vi "Instructor.vi"() -> ()   [LabVIEW 2017]
uses:
  <vilib>/Analysis/baseanly.llb/Mean (DBL).vi
  <vilib>/Utility/file.llb/Read Delimited Spreadsheet (DBL).vi
  <vilib>/Analysis/NI_AALBase.lvlib
panel:
  in  "TCHXActive":bool
  in  "PowerActive":bool
  in  "CTAHActive":bool
  in  "PumpActive":bool
  in  "ACTIVATE - TCHX_S":bool
  in  "ACTIVATE - PUMP_S":bool
  in  "ACTIVATE - CTAH_S":bool
  in  "Power Output On_S":bool
  in  "TCHXFreq_S":sgl format="%#.1f"
  in  "TCHXFreq":bool
  in  "Power_S":sgl format="%#.1f"
  in  "Power":bool
  in  "CTAHFreq_S":sgl format="%#.1f"
  in  "CTAHFreq":bool
  in  "PumpFreq_S":sgl format="%#.1f"
  in  "PumpFreq":bool
  out "W":sgl format="%.1f"
  out "S":sgl format="%.1f"
  out "E":sgl format="%.1f"
  out "N":sgl format="%.1f"
  out "SW":sgl format="%.1f"
  out "SE":sgl format="%.1f"
  out "N":sgl format="%.1f"
  out "Server Connection":bool
  out "Numeric":i32
  in  "B66":bool
  in  "W67":bool
  in  "B60":bool
  in  "W61":bool
  in  "B65":bool
  in  "W64":bool
  in  "B21":bool
  in  "W20":bool
  in  "B23":bool
  in  "W22":bool
  in  "B63":bool
  in  "W62":bool
  in  "A01":bool
  in  "A02":bool
  in  "W24":bool
  in  "B25":bool
  in  "W26":bool
  in  "B27":bool
  in  "B12":bool
  in  "W13":bool
  in  "C11":bool
  in  "C10":bool
  in  "S13":bool
  in  "S11":bool
  in  "S10":bool
  in  "W35":bool
  in  "B34":bool
  in  "B43":bool
  in  "W42":bool
  in  "W40":bool
  in  "B41":bool
  in  "W33":bool
  in  "B32":bool
  in  "W31":bool
  in  "B30":bool
  in  "W10":bool
  in  "B11":bool
  in  "B29":bool
  in  "W28":bool
  in  "Spoof Enabled":bool
  in  "Stop Instructor":bool
  in  "BT-63_S":sgl format="%.1g"
  in  "WT-35_S":sgl format="%.1g"
  in  "BT-34_S":sgl format="%.1g"
  in  "ST-13_S":sgl format="%.1g"
  in  "ST-11_S":sgl format="%.1g"
  in  "ST-10_S":sgl format="%.1g"
  in  "BT-29_S":sgl format="%.1g"
  in  "BT-60_S":sgl format="%.1g"
  in  "AT-02_S":sgl format="%.1g"
  in  "AT-01_S":sgl format="%.1g"
  in  "BT-30_S":sgl format="%.1g"
  in  "BT-66_S":sgl format="%.1g"
  in  "BT-65_S":sgl format="%.1g"
  in  "BT-21_S":sgl format="%.1g"
  in  "BT-23_S":sgl format="%.1g"
  in  "BT-25_S":sgl format="%.1g"
  in  "BT-27_S":sgl format="%.1g"
  in  "BT-32_S":sgl format="%.1g"
  in  "BT-43_S":sgl format="%.1g"
  in  "BT-41_S":sgl format="%.1g"
  in  "WT-67_S":sgl format="%.1g"
  in  "WT-61_S":sgl format="%.1g"
  in  "WT-64_S":sgl format="%.1g"
  in  "WT-62_S":sgl format="%.1g"
  in  "WT-20_S":sgl format="%.1g"
  in  "WT-22_S":sgl format="%.1g"
  in  "WT-33_S":sgl format="%.1g"
  in  "WT-24_S":sgl format="%.1g"
  in  "WT-26_S":sgl format="%.1g"
  in  "WT-28_S":sgl format="%.1g"
  in  "WT-42_S":sgl format="%.1g"
  in  "WT-40_S":sgl format="%.1g"
  in  "WT-31_S":sgl format="%.1g"
  in  "BT-12_S":sgl format="%.1g"
  in  "BT-11_S":sgl format="%.1g"
  in  "WT-10_S":sgl format="%.1g"
  in  "CX-11_S":sgl format="%.1g"
  in  "CX-10_S":sgl format="%.1g"
  out "DRACS Flow\n\n\nFM-60 [kg/s]":sgl format="%.3f"
  out "Primary Flow\n\n\nFM-40 [kg/s]":sgl format="%.3f"
  out "Bypass Flow\n\n\nFM-30 [kg/s]":sgl format="%.3f"
  out "DHX Primary Flow\n\n\nFM-20 [kg/s]":sgl format="%.3f"
  in  "ACTIVATE - PUMP":bool
  in  "ACTIVATE - TCHX":bool
  in  "ACTIVATE - CTAH":bool
  in  "Shutdown":bool
  in  "Power Output On":bool
  out "AT-02":sgl format="%.1g"
  out "AT-01":sgl format="%.1g"
  out "ST-13":sgl format="%.1f"
  out "ST-11":sgl format="%.1f"
  out "ST-10":sgl format="%.1f"
  out "WT-67":sgl format="%.1f"
  out "BT-66":sgl format="%.1f"
  out "BT-65":sgl format="%.1f"
  out "WT-64":sgl format="%.1f"
  out "BT-63":sgl format="%.1f"
  out "WT-62":sgl format="%.1f"
  out "WT-61":sgl format="%.1f"
  out "BT-60":sgl format="%.1f"
  out "BT-43":sgl format="%.1g"
  out "WT-42":sgl format="%.1g"
  out "BT-41":sgl format="%.1g"
  out "WT-40":sgl format="%.1g"
  out "WT-35":sgl format="%.1g"
  out "BT-34":sgl format="%.1g"
  out "WT-33":sgl format="%.1g"
  out "BT-32":sgl format="%.1g"
  out "WT-31":sgl format="%.1g"
  out "BT-30":sgl format="%.1g"
  out "BT-29":sgl format="%.1f"
  out "WT-28":sgl format="%.1f"
  out "BT-27":sgl format="%.1f"
  out "WT-26":sgl format="%.1f"
  out "BT-25":sgl format="%.1f"
  out "WT-24":sgl format="%.1f"
  out "BT-23":sgl format="%.1f"
  out "WT-22":sgl format="%.1f"
  out "BT-21":sgl format="%.1f"
  out "WT-20":sgl format="%.1f"
  out "CX-11":sgl format="%.1g"
  out "CX-10":sgl format="%.1g"
  out "WT-13":sgl format="%.1g"
  out "BT-12":sgl format="%.1g"
  out "BT-11":sgl format="%.1g"
  out "WT-10":sgl format="%.1g"
  in  "Desired Power [W]":dbl
  out "Power [W]":sgl(slide) caption="Power Output [W]" scale=0.0..10000.0
  out "Frequency [Hz]":sgl(knob) scale=0.0..45.0
  out "Frequency [Hz] 3":sgl(slide) scale=0.0..60.0
  out "Frequency [Hz]":sgl(slide) scale=0.0..60.0
  in  "WT-13_S":sgl format="%.1g"
  out "Power Output":sgl(graph)
  in  "Flow Data?":bool=TRUE
  out "System Safe":bool
  in  "Exit Profile":bool
  in  "Select Operation Mode":T1(ring) caption="Select Operation Mode2"
  out "System Time [s]":sgl format="%#.1f"
  out "System Loop Time (ms)":u32
  in  "Load Power Profile":bool
  in  "Dyn. Power Profile File":path
  out "CTAH Temperatures":cluster{"CTAH Outlet":dbl, "CTAH Inlet":dbl}(graph)
  out "CTAH Outlet":dbl format="%0.2f"
  out "CTAH Inlet":dbl format="%0.2f"
  out "Core Temperatures":cluster{"Heater Inlet":dbl, "Heater Outlet":dbl}(graph)
  out "Heater Outlet":dbl format="%0.2f"
  out "Heater Inlet":dbl format="%0.2f"
  out "Profile Step":i32
  out "Power Input Signal [W]":dbl
  out "Output Current 2 [A]":dbl
  out "Output Voltage 2 [V]":dbl
  out "Output Current 1 [A]":dbl
  out "Output Voltage 1 [V]":dbl
  out "Loop Period [ms]":i64
  in  "Pump Operation Mode":i32(listbox)
  in  "TCHX Operation Mode":i32(listbox)
  in  "VFD Stop":bool
  in  "CTAH Operation Mode":i32(listbox)
  # "System Analytics"
  # "DRACS"
  # "PRIMARY"
  # "HOT DRACS"
  # "DHX TOP"
  # "TCHX"
  # "HOT LEG"
  # "DHX"
  # "COLD DRACS"
  # "ST-14"
  # "BYPASS"
  # "CTAH"
  # "ST-12"
  # "DHX BOTTOM"
  # "HEATER"
  # "COLD LEG"
  # "PUMP"
  # "Action Log"
  # "Action Log Box"
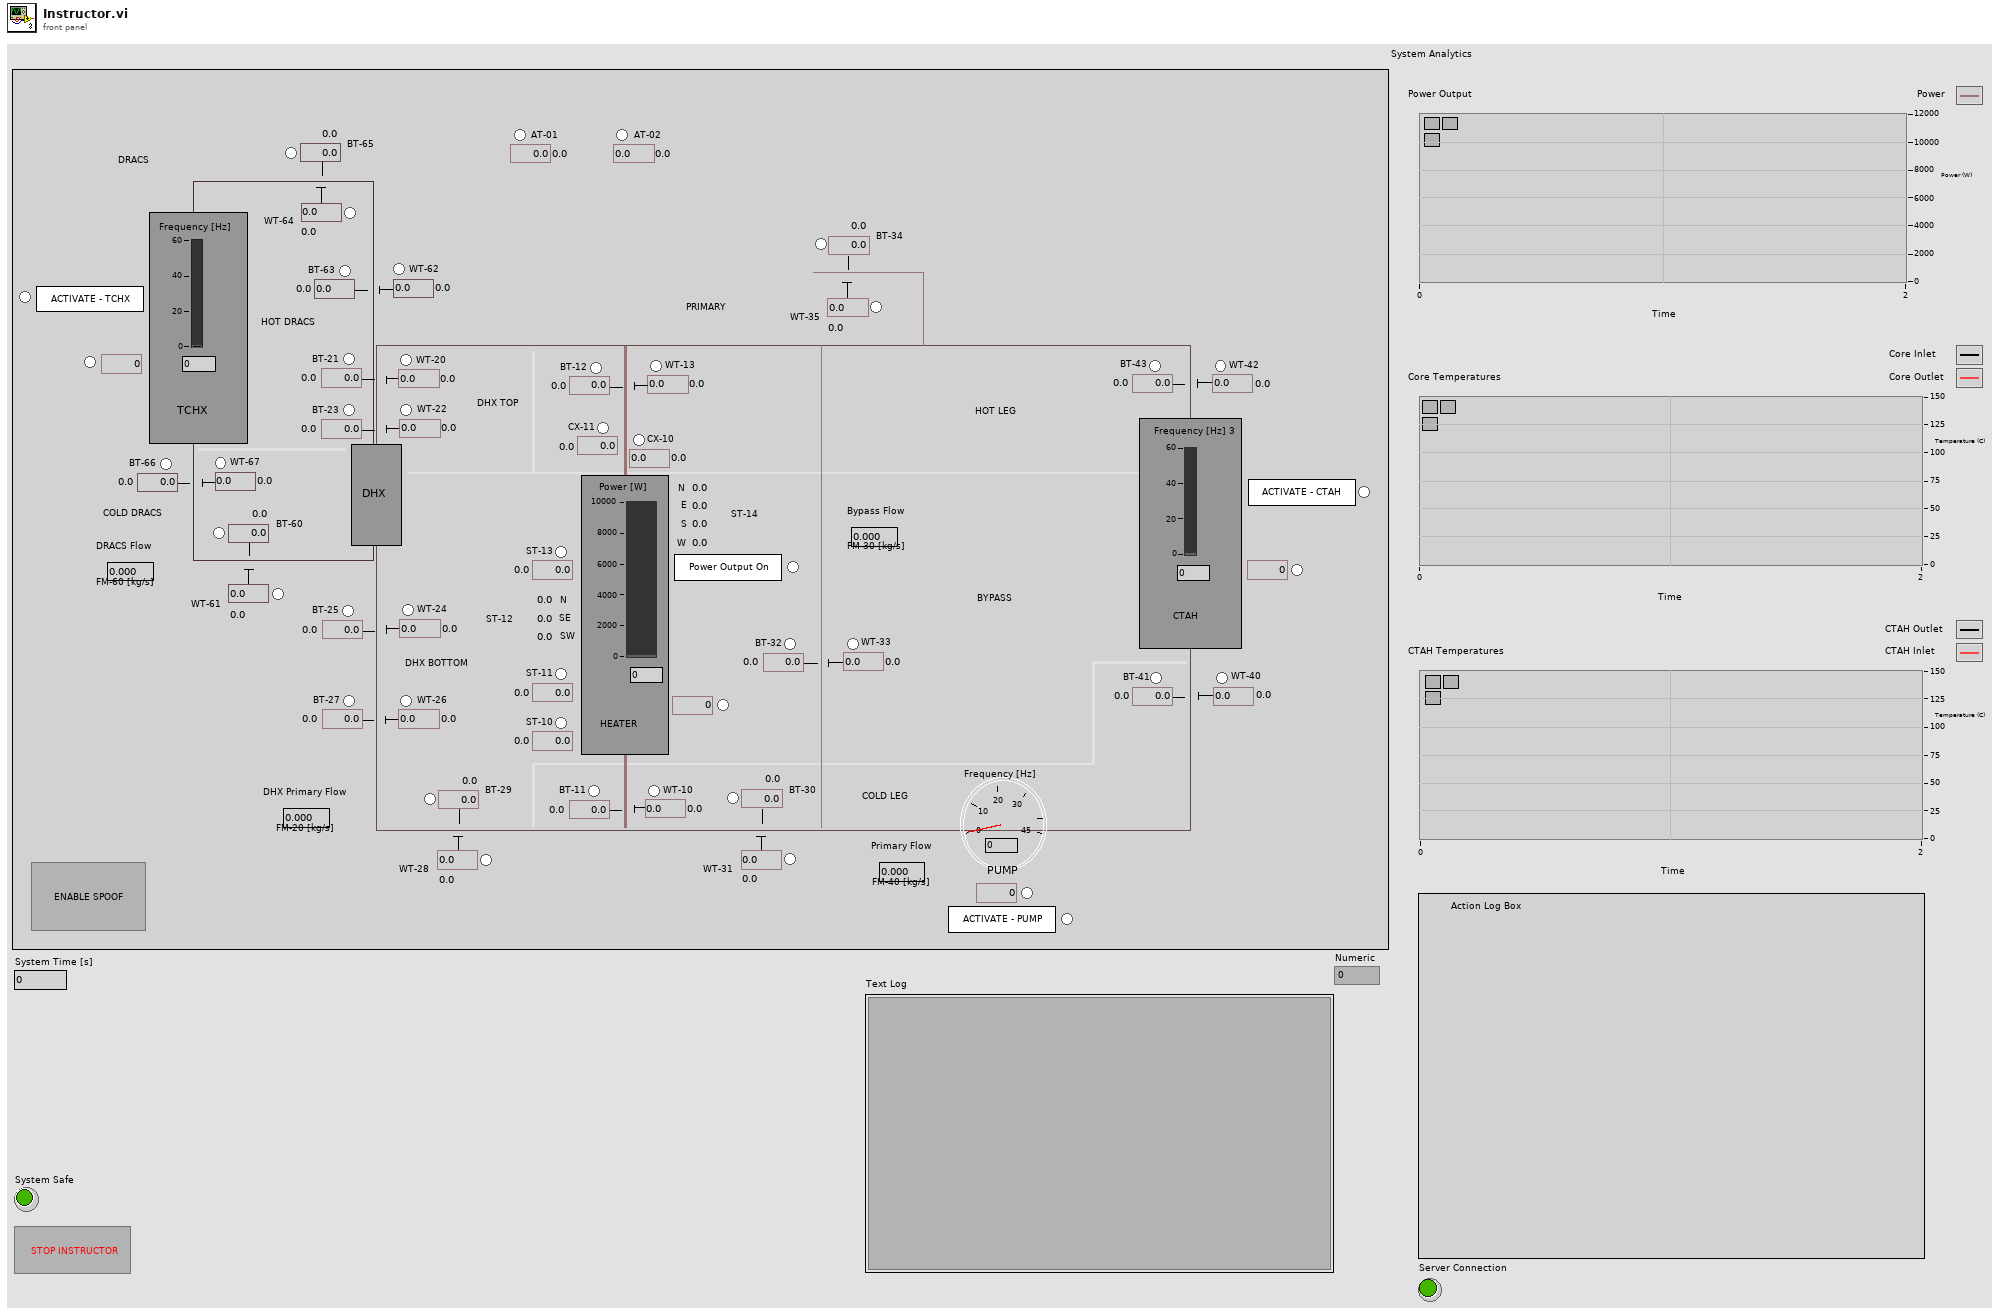
[diagram p1: front panel]
types:
  T1 = enum16{"Resistance Feedback", "Power Profile Input", "Resistance Feedback_Analog", "Power Profile Input_Analog", "Shutdown"}
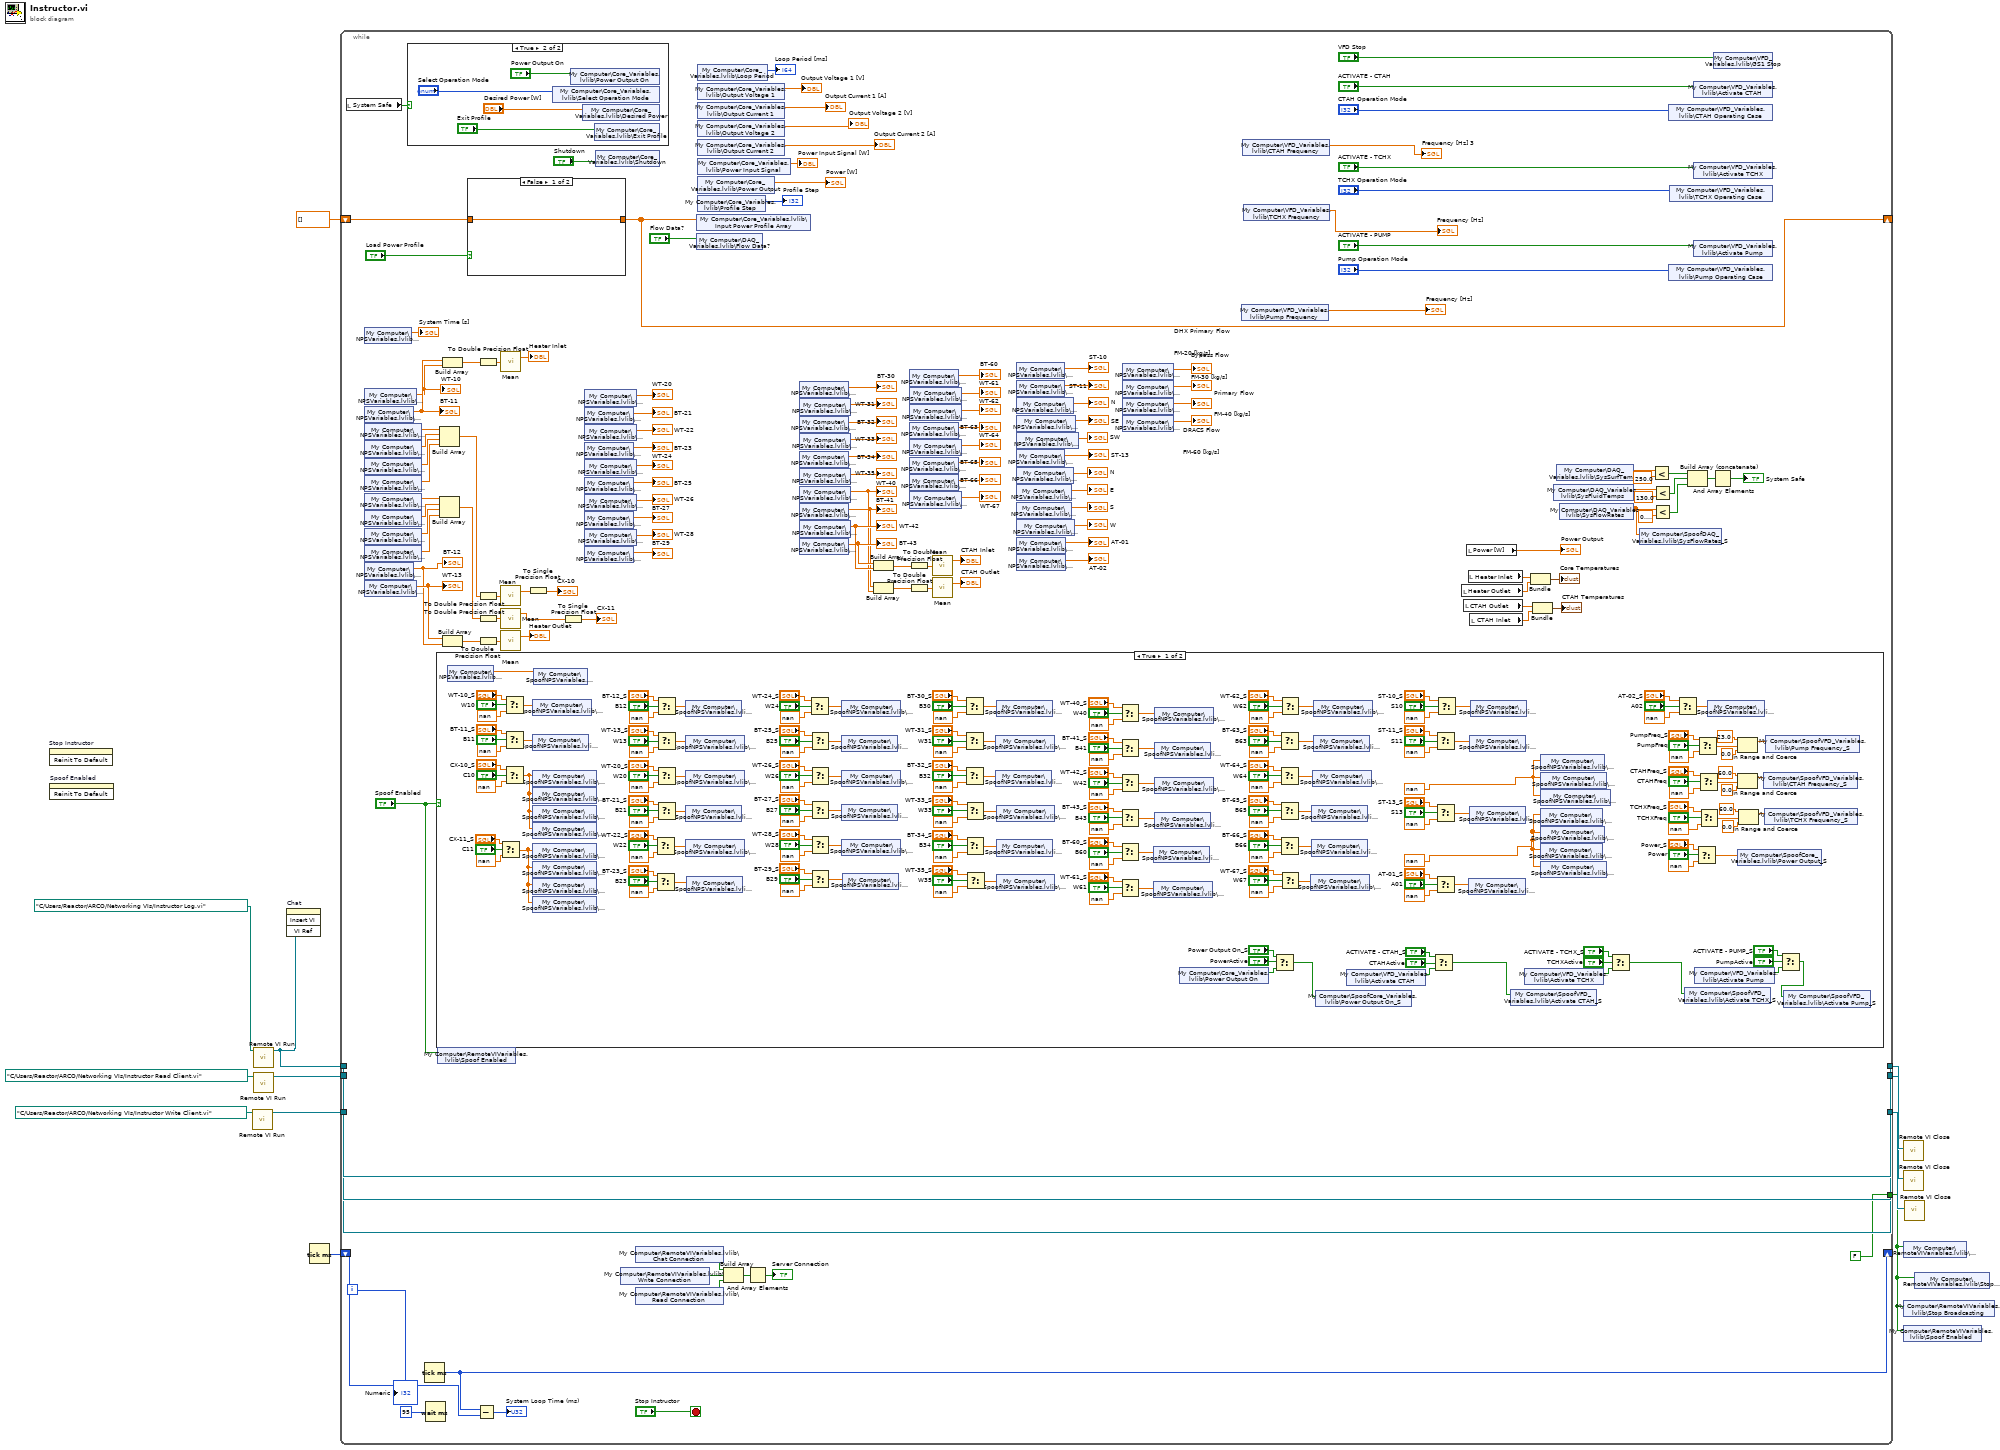
[diagram p0: block diagram]
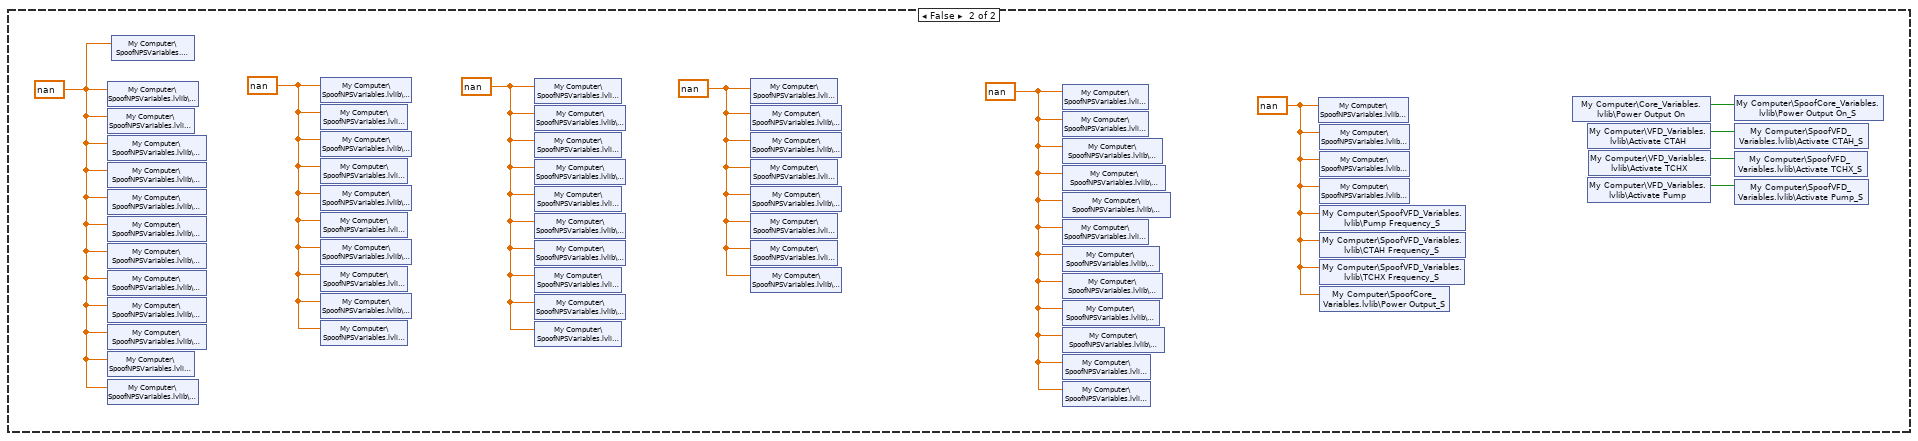
[diagram p2: hidden frame]
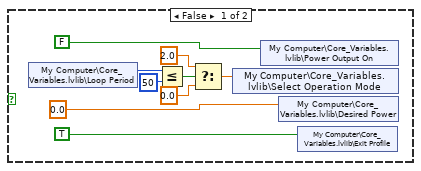
[diagram p3: hidden frame]
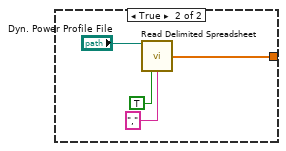
[diagram p4: hidden frame]
diagram:
  n1 = invoke on="Stop Instructor" class="Bool (strict)" method="Reinit To Default"() -> ()  [unwired: 3 in, 3 out]
  n2 = invoke on="Spoof Enabled" class="Bool (strict)" method="Reinit To Default"() -> ()  [unwired: 3 in, 3 out]
  n3 = call "Remote VI Run.vi"("VI Path"=path "C:/Users/Reactor/ARCO/Networking VIs/Instructor Write Client.vi") -> ("VI Reference"=w3:refnum<vi>)  [unwired: 10 in]
  n4 = call "Remote VI Run.vi"("VI Path"=path "C:/Users/Reactor/ARCO/Networking VIs/Instructor Log.vi" ("vi path")) -> ("VI Reference"=w9:refnum<vi>)  [unwired: 10 in]
  n5 = call "Remote VI Run.vi"("VI Path"=path "C:/Users/Reactor/ARCO/Networking VIs/Instructor Read Client.vi") -> ("VI Reference"=w7:refnum<vi>)  [unwired: 10 in]
  n6 = invoke on="Chat" class="SubPnl" method="Insert VI"("VI Ref"=w9) -> ()  [unwired: 3 in, 4 out]
  n7 = Tick Count (ms)() -> (millisecond timer value=w11:u32)
  n8 = while {
    shift-right: [w65] -> _
    shift-left: dbl[] [] ("Input Power Profile Array") -> [w66]
    shift-right: [w63] -> _
    shift-left: w11 -> [w64]
    tunnel: w9 -> [w34]
    tunnel: w7 -> [w33]
    tunnel: [w34] -> w6
    tunnel: [w33] -> w5
    tunnel: w3 -> [w32]
    tunnel: [w32] -> w2
    tunnel: [FALSE] -> w1
    i -> [w30]
    stop <- "Stop Instructor" stop-if-true
    n9 = local read "System Safe"() -> (w51:bool)
    n10 = shared-variable "My Computer\\NPSVariables.lvlib\\Time"() -> (→"System Time [s]":sgl)  [unwired: 1 in, 1 out]
    n11 = shared-variable "My Computer\\NPSVariables.lvlib\\WT-10"() -> (w41:sgl)  [unwired: 1 in, 1 out]
    "WT-10" <- w41
    n12 = shared-variable "My Computer\\NPSVariables.lvlib\\BT-11"() -> (w45:sgl)  [unwired: 1 in, 1 out]
    "BT-11" <- w45
    n13 = shared-variable "My Computer\\NPSVariables.lvlib\\CX-10-1"() -> (w131:sgl)  [unwired: 1 in, 1 out]
    n14 = shared-variable "My Computer\\NPSVariables.lvlib\\CX-10-2"() -> (w130:sgl)  [unwired: 1 in, 1 out]
    n15 = shared-variable "My Computer\\NPSVariables.lvlib\\CX-10-3"() -> (w129:sgl)  [unwired: 1 in, 1 out]
    n16 = shared-variable "My Computer\\NPSVariables.lvlib\\CX-10-4"() -> (w128:sgl)  [unwired: 1 in, 1 out]
    n17 = shared-variable "My Computer\\NPSVariables.lvlib\\CX-11-1"() -> (w124:sgl)  [unwired: 1 in, 1 out]
    n18 = shared-variable "My Computer\\NPSVariables.lvlib\\CX-11-2"() -> (w123:sgl)  [unwired: 1 in, 1 out]
    n19 = shared-variable "My Computer\\NPSVariables.lvlib\\CX-11-3"() -> (w122:sgl)  [unwired: 1 in, 1 out]
    n20 = shared-variable "My Computer\\NPSVariables.lvlib\\CX-11-4"() -> (w121:sgl)  [unwired: 1 in, 1 out]
    n21 = shared-variable "My Computer\\NPSVariables.lvlib\\BT-12"() -> (w44:sgl)  [unwired: 1 in, 1 out]
    "BT-12" <- w44
    n22 = shared-variable "My Computer\\NPSVariables.lvlib\\WT-13"() -> (w88:sgl)  [unwired: 1 in, 1 out]
    "WT-13" <- w88
    n23 = case shown="True" w51 {
      frame False {
        n24 = shared-variable "My Computer\\Core_Variables.lvlib\\Loop Period"() -> (w362:i64)  [unwired: 1 in, 1 out]
        n25 = Less Or Equal?(x=w362, y=i64 50) -> (x <= y?=w363:bool)
        n26 = Select(t=2.0, s=w363, f=0.0) -> (s? t:f=w358:dbl)
        n27 = shared-variable "My Computer\\Core_Variables.lvlib\\Select Operation Mode"(w358) -> ()  [unwired: 1 in, 1 out]
        n28 = shared-variable "My Computer\\Core_Variables.lvlib\\Power Output On"(FALSE ("Power Output On")) -> ()  [unwired: 1 in, 1 out]
        n29 = shared-variable "My Computer\\Core_Variables.lvlib\\Desired Power"(0.0 ("Desired Power")) -> ()  [unwired: 1 in, 1 out]
        n30 = shared-variable "My Computer\\Core_Variables.lvlib\\Exit Profile"(TRUE ("Exit Profile")) -> ()  [unwired: 1 in, 1 out]
      }
      frame True {
        n31 = shared-variable "My Computer\\Core_Variables.lvlib\\Select Operation Mode"("Select Operation Mode") -> ()  [unwired: 1 in, 1 out]
        n32 = shared-variable "My Computer\\Core_Variables.lvlib\\Power Output On"("Power Output On") -> ()  [unwired: 1 in, 1 out]
        n33 = shared-variable "My Computer\\Core_Variables.lvlib\\Desired Power"("Desired Power [W]") -> ()  [unwired: 1 in, 1 out]
        n34 = shared-variable "My Computer\\Core_Variables.lvlib\\Exit Profile"("Exit Profile") -> ()  [unwired: 1 in, 1 out]
      }
    }
    n35 = Tick Count (ms)() -> (millisecond timer value=w63:u32)
    n36 = Wait (ms)(milliseconds to wait=u32 95) -> ()  [unwired: 1 out]
    n37 = case shown="True" "Spoof Enabled" {
      frame True {
        w189 = sgl nan
        w190 = sgl nan
        n38 = shared-variable "My Computer\\NPSVariables.lvlib\\Time"() -> (w191:sgl)  [unwired: 1 in, 1 out]
        n39 = Select(t="CX-11_S", s="C11", f=sgl nan) -> (s? t:f=w332:sgl)
        n40 = Select(t="WT-10_S", s="W10", f=sgl nan) -> (s? t:f=w344:sgl)
        n41 = Select(t="BT-11_S", s="B11", f=sgl nan) -> (s? t:f=w340:sgl)
        n42 = Select(t="CX-10_S", s="C10", f=sgl nan) -> (s? t:f=w336:sgl)
        n43 = shared-variable "My Computer\\SpoofNPSVariables.lvlib\\WT-10_S"(w344) -> ()  [unwired: 1 in, 1 out]
        n44 = shared-variable "My Computer\\SpoofNPSVariables.lvlib\\BT-11_S"(w340) -> ()  [unwired: 1 in, 1 out]
        n45 = shared-variable "My Computer\\SpoofNPSVariables.lvlib\\CX-10-1_S"(w336) -> ()  [unwired: 1 in, 1 out]
        n46 = shared-variable "My Computer\\SpoofNPSVariables.lvlib\\CX-10-2_S"(w336) -> ()  [unwired: 1 in, 1 out]
        n47 = shared-variable "My Computer\\SpoofNPSVariables.lvlib\\CX-10-3_S"(w336) -> ()  [unwired: 1 in, 1 out]
        n48 = shared-variable "My Computer\\SpoofNPSVariables.lvlib\\CX-10-4_S"(w336) -> ()  [unwired: 1 in, 1 out]
        n49 = shared-variable "My Computer\\SpoofNPSVariables.lvlib\\CX-11-1_S"(w332) -> ()  [unwired: 1 in, 1 out]
        n50 = shared-variable "My Computer\\SpoofNPSVariables.lvlib\\CX-11-2_S"(w332) -> ()  [unwired: 1 in, 1 out]
        n51 = shared-variable "My Computer\\SpoofNPSVariables.lvlib\\CX-11-3_S"(w332) -> ()  [unwired: 1 in, 1 out]
        n52 = shared-variable "My Computer\\SpoofNPSVariables.lvlib\\CX-11-4_S"(w332) -> ()  [unwired: 1 in, 1 out]
        n53 = shared-variable "My Computer\\SpoofNPSVariables.lvlib\\Time_S"(w191) -> ()  [unwired: 1 in, 1 out]
        n54 = Select(t="WT-22_S", s="W22", f=sgl nan) -> (s? t:f=w312:sgl)
        n55 = Select(t="BT-23_S", s="B23", f=sgl nan) -> (s? t:f=w308:sgl)
        n56 = Select(t="BT-12_S", s="B12", f=sgl nan) -> (s? t:f=w328:sgl)
        n57 = Select(t="WT-13_S", s="W13", f=sgl nan) -> (s? t:f=w324:sgl)
        n58 = Select(t="WT-20_S", s="W20", f=sgl nan) -> (s? t:f=w320:sgl)
        n59 = Select(t="BT-21_S", s="B21", f=sgl nan) -> (s? t:f=w316:sgl)
        n60 = shared-variable "My Computer\\SpoofNPSVariables.lvlib\\BT-12_S"(w328) -> ()  [unwired: 1 in, 1 out]
        n61 = shared-variable "My Computer\\SpoofNPSVariables.lvlib\\WT-13_S"(w324) -> ()  [unwired: 1 in, 1 out]
        n62 = shared-variable "My Computer\\SpoofNPSVariables.lvlib\\WT-20_S"(w320) -> ()  [unwired: 1 in, 1 out]
        n63 = shared-variable "My Computer\\SpoofNPSVariables.lvlib\\BT-21_S"(w316) -> ()  [unwired: 1 in, 1 out]
        n64 = shared-variable "My Computer\\SpoofNPSVariables.lvlib\\WT-22_S"(w312) -> ()  [unwired: 1 in, 1 out]
        n65 = shared-variable "My Computer\\SpoofNPSVariables.lvlib\\BT-23_S"(w308) -> ()  [unwired: 1 in, 1 out]
        n66 = Select(t="WT-24_S", s="W24", f=sgl nan) -> (s? t:f=w304:sgl)
        n67 = Select(t="BT-25_S", s="B25", f=sgl nan) -> (s? t:f=w300:sgl)
        n68 = Select(t="WT-26_S", s="W26", f=sgl nan) -> (s? t:f=w296:sgl)
        n69 = Select(t="BT-27_S", s="B27", f=sgl nan) -> (s? t:f=w292:sgl)
        n70 = Select(t="WT-28_S", s="W28", f=sgl nan) -> (s? t:f=w288:sgl)
        n71 = Select(t="BT-29_S", s="B29", f=sgl nan) -> (s? t:f=w284:sgl)
        n72 = shared-variable "My Computer\\SpoofNPSVariables.lvlib\\WT-24_S"(w304) -> ()  [unwired: 1 in, 1 out]
        n73 = shared-variable "My Computer\\SpoofNPSVariables.lvlib\\BT-25_S"(w300) -> ()  [unwired: 1 in, 1 out]
        n74 = shared-variable "My Computer\\SpoofNPSVariables.lvlib\\WT-26_S"(w296) -> ()  [unwired: 1 in, 1 out]
        n75 = shared-variable "My Computer\\SpoofNPSVariables.lvlib\\BT-27_S"(w292) -> ()  [unwired: 1 in, 1 out]
        n76 = shared-variable "My Computer\\SpoofNPSVariables.lvlib\\WT-28_S"(w288) -> ()  [unwired: 1 in, 1 out]
        n77 = shared-variable "My Computer\\SpoofNPSVariables.lvlib\\BT-29_S"(w284) -> ()  [unwired: 1 in, 1 out]
        n78 = Select(t="BT-30_S", s="B30", f=sgl nan) -> (s? t:f=w280:sgl)
        n79 = Select(t="WT-31_S", s="W31", f=sgl nan) -> (s? t:f=w276:sgl)
        n80 = Select(t="BT-32_S", s="B32", f=sgl nan) -> (s? t:f=w272:sgl)
        n81 = Select(t="WT-33_S", s="W33", f=sgl nan) -> (s? t:f=w268:sgl)
        n82 = Select(t="BT-34_S", s="B34", f=sgl nan) -> (s? t:f=w264:sgl)
        n83 = Select(t="WT-35_S", s="W35", f=sgl nan) -> (s? t:f=w260:sgl)
        n84 = shared-variable "My Computer\\SpoofNPSVariables.lvlib\\WT-31_S"(w276) -> ()  [unwired: 1 in, 1 out]
        n85 = shared-variable "My Computer\\SpoofNPSVariables.lvlib\\BT-32_S"(w272) -> ()  [unwired: 1 in, 1 out]
        n86 = shared-variable "My Computer\\SpoofNPSVariables.lvlib\\BT-30_S"(w280) -> ()  [unwired: 1 in, 1 out]
        n87 = shared-variable "My Computer\\SpoofNPSVariables.lvlib\\WT-33_S"(w268) -> ()  [unwired: 1 in, 1 out]
        n88 = shared-variable "My Computer\\SpoofNPSVariables.lvlib\\BT-34_S"(w264) -> ()  [unwired: 1 in, 1 out]
        n89 = shared-variable "My Computer\\SpoofNPSVariables.lvlib\\WT-35_S"(w260) -> ()  [unwired: 1 in, 1 out]
        n90 = Select(t="WT-40_S", s="W40", f=sgl nan) -> (s? t:f=w256:sgl)
        n91 = Select(t="BT-41_S", s="B41", f=sgl nan) -> (s? t:f=w252:sgl)
        n92 = Select(t="WT-42_S", s="W42", f=sgl nan) -> (s? t:f=w248:sgl)
        n93 = Select(t="BT-43_S", s="B43", f=sgl nan) -> (s? t:f=w244:sgl)
        n94 = Select(t="BT-60_S", s="B60", f=sgl nan) -> (s? t:f=w240:sgl)
        n95 = Select(t="WT-61_S", s="W61", f=sgl nan) -> (s? t:f=w236:sgl)
        n96 = shared-variable "My Computer\\SpoofNPSVariables.lvlib\\BT-60_S"(w240) -> ()  [unwired: 1 in, 1 out]
        n97 = shared-variable "My Computer\\SpoofNPSVariables.lvlib\\WT-61_S"(w236) -> ()  [unwired: 1 in, 1 out]
        n98 = shared-variable "My Computer\\SpoofNPSVariables.lvlib\\BT-41_S"(w252) -> ()  [unwired: 1 in, 1 out]
        n99 = shared-variable "My Computer\\SpoofNPSVariables.lvlib\\WT-42_S"(w248) -> ()  [unwired: 1 in, 1 out]
        n100 = shared-variable "My Computer\\SpoofNPSVariables.lvlib\\BT-43_S"(w244) -> ()  [unwired: 1 in, 1 out]
        n101 = shared-variable "My Computer\\SpoofNPSVariables.lvlib\\WT-40_S"(w256) -> ()  [unwired: 1 in, 1 out]
        n102 = shared-variable "My Computer\\Core_Variables.lvlib\\Power Output On"() -> (w161:bool)  [unwired: 1 in, 1 out]
        n103 = Select(t="Power Output On_S", s="PowerActive", f=w161) -> (s? t:f=w151:bool)
        n104 = Select(t="BT-63_S", s="B63", f=sgl nan) -> (s? t:f=w228:sgl)
        n105 = Select(t="WT-64_S", s="W64", f=sgl nan) -> (s? t:f=w224:sgl)
        n106 = Select(t="BT-65_S", s="B65", f=sgl nan) -> (s? t:f=w220:sgl)
        n107 = Select(t="BT-66_S", s="B66", f=sgl nan) -> (s? t:f=w216:sgl)
        n108 = Select(t="WT-62_S", s="W62", f=sgl nan) -> (s? t:f=w232:sgl)
        n109 = Select(t="WT-67_S", s="W67", f=sgl nan) -> (s? t:f=w212:sgl)
        n110 = shared-variable "My Computer\\SpoofNPSVariables.lvlib\\WT-67_S"(w212) -> ()  [unwired: 1 in, 1 out]
        n111 = shared-variable "My Computer\\SpoofNPSVariables.lvlib\\BT-66_S"(w216) -> ()  [unwired: 1 in, 1 out]
        n112 = shared-variable "My Computer\\SpoofNPSVariables.lvlib\\BT-65_S"(w220) -> ()  [unwired: 1 in, 1 out]
        n113 = shared-variable "My Computer\\SpoofNPSVariables.lvlib\\WT-64_S"(w224) -> ()  [unwired: 1 in, 1 out]
        n114 = shared-variable "My Computer\\SpoofNPSVariables.lvlib\\BT-63_S"(w228) -> ()  [unwired: 1 in, 1 out]
        n115 = shared-variable "My Computer\\SpoofNPSVariables.lvlib\\WT-62_S"(w232) -> ()  [unwired: 1 in, 1 out]
        n116 = shared-variable "My Computer\\SpoofCore_Variables.lvlib\\Power Output On_S"(w151) -> ()  [unwired: 1 in, 1 out]
        n117 = shared-variable "My Computer\\VFD_Variables.lvlib\\Activate CTAH"() -> (w158:bool)  [unwired: 1 in, 1 out]
        n118 = Select(t="ACTIVATE - CTAH_S", s="CTAHActive", f=w158) -> (s? t:f=w150:bool)
        n119 = Select(t="ST-11_S", s="S11", f=sgl nan) -> (s? t:f=w204:sgl)
        n120 = Select(t="ST-13_S", s="S13", f=sgl nan) -> (s? t:f=w200:sgl)
        n121 = Select(t="AT-01_S", s="A01", f=sgl nan) -> (s? t:f=w196:sgl)
        n122 = Select(t="ST-10_S", s="S10", f=sgl nan) -> (s? t:f=w208:sgl)
        n123 = shared-variable "My Computer\\SpoofNPSVariables.lvlib\\AT-01_S"(w196) -> ()  [unwired: 1 in, 1 out]
        n124 = shared-variable "My Computer\\SpoofNPSVariables.lvlib\\ST-11_S"(w204) -> ()  [unwired: 1 in, 1 out]
        n125 = shared-variable "My Computer\\SpoofNPSVariables.lvlib\\ST-13_S"(w200) -> ()  [unwired: 1 in, 1 out]
        n126 = shared-variable "My Computer\\SpoofNPSVariables.lvlib\\ST-10_S"(w208) -> ()  [unwired: 1 in, 1 out]
        n127 = shared-variable "My Computer\\SpoofVFD_Variables.lvlib\\Activate CTAH_S"(w150) -> ()  [unwired: 1 in, 1 out]
        n128 = shared-variable "My Computer\\VFD_Variables.lvlib\\Activate TCHX"() -> (w155:bool)  [unwired: 1 in, 1 out]
        n129 = shared-variable "My Computer\\SpoofNPSVariables.lvlib\\ST-12-N_S"(w190) -> ()  [unwired: 1 in, 1 out]
        n130 = shared-variable "My Computer\\SpoofNPSVariables.lvlib\\ST-12-SE_S"(w190) -> ()  [unwired: 1 in, 1 out]
        n131 = shared-variable "My Computer\\SpoofNPSVariables.lvlib\\ST-12-SW_S"(w190) -> ()  [unwired: 1 in, 1 out]
        n132 = shared-variable "My Computer\\SpoofNPSVariables.lvlib\\ST-14-E_S"(w189) -> ()  [unwired: 1 in, 1 out]
        n133 = shared-variable "My Computer\\SpoofNPSVariables.lvlib\\ST-14-N_S"(w189) -> ()  [unwired: 1 in, 1 out]
        n134 = shared-variable "My Computer\\SpoofNPSVariables.lvlib\\ST-14-S_S"(w189) -> ()  [unwired: 1 in, 1 out]
        n135 = shared-variable "My Computer\\SpoofNPSVariables.lvlib\\ST-14-W_S"(w189) -> ()  [unwired: 1 in, 1 out]
        n136 = Select(t="ACTIVATE - TCHX_S", s="TCHXActive", f=w155) -> (s? t:f=w148:bool)
        n137 = Select(t="AT-02_S", s="A02", f=sgl nan) -> (s? t:f=w192:sgl)
        n138 = shared-variable "My Computer\\SpoofVFD_Variables.lvlib\\Activate TCHX_S"(w148) -> ()  [unwired: 1 in, 1 out]
        n139 = shared-variable "My Computer\\VFD_Variables.lvlib\\Activate Pump"() -> (w152:bool)  [unwired: 1 in, 1 out]
        n140 = Select(t="Power_S", s="Power", f=sgl nan) -> (s? t:f=w164:sgl)
        n141 = Select(t="PumpFreq_S", s="PumpFreq", f=sgl nan) -> (s? t:f=w183:sgl)
        n142 = Select(t="CTAHFreq_S", s="CTAHFreq", f=sgl nan) -> (s? t:f=w179:sgl)
        n143 = Select(t="TCHXFreq_S", s="TCHXFreq", f=sgl nan) -> (s? t:f=w172:sgl)
        n144 = shared-variable "My Computer\\SpoofNPSVariables.lvlib\\AT-02_S"(w192) -> ()  [unwired: 1 in, 1 out]
        n145 = In Range and Coerce(upper limit=sgl 23.0, x=w183, lower limit=sgl 0.0) -> (coerced(x)=w182:sgl)  [unwired: 1 out]
        n146 = shared-variable "My Computer\\SpoofCore_Variables.lvlib\\Power Output_S"(w164) -> ()  [unwired: 1 in, 1 out]
        n147 = In Range and Coerce(upper limit=sgl 60.0, x=w179, lower limit=sgl 0.0) -> (coerced(x)=w175:sgl)  [unwired: 1 out]
        n148 = In Range and Coerce(upper limit=sgl 60.0, x=w172, lower limit=sgl 0.0) -> (coerced(x)=w168:sgl)  [unwired: 1 out]
        n149 = shared-variable "My Computer\\SpoofVFD_Variables.lvlib\\CTAH Frequency_S"(w175) -> ()  [unwired: 1 in, 1 out]
        n150 = shared-variable "My Computer\\SpoofVFD_Variables.lvlib\\TCHX Frequency_S"(w168) -> ()  [unwired: 1 in, 1 out]
        n151 = shared-variable "My Computer\\SpoofVFD_Variables.lvlib\\Pump Frequency_S"(w182) -> ()  [unwired: 1 in, 1 out]
        n152 = Select(t="ACTIVATE - PUMP_S", s="PumpActive", f=w152) -> (s? t:f=w149:bool)
        n153 = shared-variable "My Computer\\SpoofVFD_Variables.lvlib\\Activate Pump_S"(w149) -> ()  [unwired: 1 in, 1 out]
      }
      frame False {
        w352 = sgl nan
        w354 = sgl nan
        w355 = sgl nan
        w356 = sgl nan
        w357 = sgl nan
        w353 = sgl nan
        n154 = shared-variable "My Computer\\SpoofNPSVariables.lvlib\\WT-10_S"(w353) -> ()  [unwired: 1 in, 1 out]
        n155 = shared-variable "My Computer\\SpoofNPSVariables.lvlib\\BT-11_S"(w353) -> ()  [unwired: 1 in, 1 out]
        n156 = shared-variable "My Computer\\SpoofNPSVariables.lvlib\\CX-10-1_S"(w353) -> ()  [unwired: 1 in, 1 out]
        n157 = shared-variable "My Computer\\SpoofNPSVariables.lvlib\\CX-10-2_S"(w353) -> ()  [unwired: 1 in, 1 out]
        n158 = shared-variable "My Computer\\SpoofNPSVariables.lvlib\\CX-10-3_S"(w353) -> ()  [unwired: 1 in, 1 out]
        n159 = shared-variable "My Computer\\SpoofNPSVariables.lvlib\\CX-10-4_S"(w353) -> ()  [unwired: 1 in, 1 out]
        n160 = shared-variable "My Computer\\SpoofNPSVariables.lvlib\\CX-11-1_S"(w353) -> ()  [unwired: 1 in, 1 out]
        n161 = shared-variable "My Computer\\SpoofNPSVariables.lvlib\\CX-11-2_S"(w353) -> ()  [unwired: 1 in, 1 out]
        n162 = shared-variable "My Computer\\SpoofNPSVariables.lvlib\\CX-11-3_S"(w353) -> ()  [unwired: 1 in, 1 out]
        n163 = shared-variable "My Computer\\SpoofNPSVariables.lvlib\\CX-11-4_S"(w353) -> ()  [unwired: 1 in, 1 out]
        n164 = shared-variable "My Computer\\SpoofNPSVariables.lvlib\\BT-12_S"(w353) -> ()  [unwired: 1 in, 1 out]
        n165 = shared-variable "My Computer\\SpoofNPSVariables.lvlib\\WT-13_S"(w353) -> ()  [unwired: 1 in, 1 out]
        n166 = shared-variable "My Computer\\SpoofNPSVariables.lvlib\\Time_S"(w353) -> ()  [unwired: 1 in, 1 out]
        n167 = shared-variable "My Computer\\SpoofNPSVariables.lvlib\\WT-20_S"(w357) -> ()  [unwired: 1 in, 1 out]
        n168 = shared-variable "My Computer\\SpoofNPSVariables.lvlib\\BT-21_S"(w357) -> ()  [unwired: 1 in, 1 out]
        n169 = shared-variable "My Computer\\SpoofNPSVariables.lvlib\\WT-22_S"(w357) -> ()  [unwired: 1 in, 1 out]
        n170 = shared-variable "My Computer\\SpoofNPSVariables.lvlib\\BT-23_S"(w357) -> ()  [unwired: 1 in, 1 out]
        n171 = shared-variable "My Computer\\SpoofNPSVariables.lvlib\\WT-24_S"(w357) -> ()  [unwired: 1 in, 1 out]
        n172 = shared-variable "My Computer\\SpoofNPSVariables.lvlib\\BT-25_S"(w357) -> ()  [unwired: 1 in, 1 out]
        n173 = shared-variable "My Computer\\SpoofNPSVariables.lvlib\\WT-26_S"(w357) -> ()  [unwired: 1 in, 1 out]
        n174 = shared-variable "My Computer\\SpoofNPSVariables.lvlib\\BT-27_S"(w357) -> ()  [unwired: 1 in, 1 out]
        n175 = shared-variable "My Computer\\SpoofNPSVariables.lvlib\\WT-28_S"(w357) -> ()  [unwired: 1 in, 1 out]
        n176 = shared-variable "My Computer\\SpoofNPSVariables.lvlib\\BT-29_S"(w357) -> ()  [unwired: 1 in, 1 out]
        n177 = shared-variable "My Computer\\SpoofNPSVariables.lvlib\\BT-30_S"(w356) -> ()  [unwired: 1 in, 1 out]
        n178 = shared-variable "My Computer\\SpoofNPSVariables.lvlib\\WT-31_S"(w356) -> ()  [unwired: 1 in, 1 out]
        n179 = shared-variable "My Computer\\SpoofNPSVariables.lvlib\\BT-32_S"(w356) -> ()  [unwired: 1 in, 1 out]
        n180 = shared-variable "My Computer\\SpoofNPSVariables.lvlib\\WT-33_S"(w356) -> ()  [unwired: 1 in, 1 out]
        n181 = shared-variable "My Computer\\SpoofNPSVariables.lvlib\\BT-34_S"(w356) -> ()  [unwired: 1 in, 1 out]
        n182 = shared-variable "My Computer\\SpoofNPSVariables.lvlib\\WT-35_S"(w356) -> ()  [unwired: 1 in, 1 out]
        n183 = shared-variable "My Computer\\SpoofNPSVariables.lvlib\\WT-40_S"(w356) -> ()  [unwired: 1 in, 1 out]
        n184 = shared-variable "My Computer\\SpoofNPSVariables.lvlib\\BT-41_S"(w356) -> ()  [unwired: 1 in, 1 out]
        n185 = shared-variable "My Computer\\SpoofNPSVariables.lvlib\\WT-42_S"(w356) -> ()  [unwired: 1 in, 1 out]
        n186 = shared-variable "My Computer\\SpoofNPSVariables.lvlib\\BT-43_S"(w356) -> ()  [unwired: 1 in, 1 out]
        n187 = shared-variable "My Computer\\SpoofNPSVariables.lvlib\\BT-60_S"(w355) -> ()  [unwired: 1 in, 1 out]
        n188 = shared-variable "My Computer\\SpoofNPSVariables.lvlib\\WT-61_S"(w355) -> ()  [unwired: 1 in, 1 out]
        n189 = shared-variable "My Computer\\SpoofNPSVariables.lvlib\\WT-62_S"(w355) -> ()  [unwired: 1 in, 1 out]
        n190 = shared-variable "My Computer\\SpoofNPSVariables.lvlib\\BT-63_S"(w355) -> ()  [unwired: 1 in, 1 out]
        n191 = shared-variable "My Computer\\SpoofNPSVariables.lvlib\\WT-64_S"(w355) -> ()  [unwired: 1 in, 1 out]
        n192 = shared-variable "My Computer\\SpoofNPSVariables.lvlib\\BT-65_S"(w355) -> ()  [unwired: 1 in, 1 out]
        n193 = shared-variable "My Computer\\SpoofNPSVariables.lvlib\\BT-66_S"(w355) -> ()  [unwired: 1 in, 1 out]
        n194 = shared-variable "My Computer\\SpoofNPSVariables.lvlib\\WT-67_S"(w355) -> ()  [unwired: 1 in, 1 out]
        n195 = shared-variable "My Computer\\SpoofNPSVariables.lvlib\\ST-10_S"(w354) -> ()  [unwired: 1 in, 1 out]
        n196 = shared-variable "My Computer\\SpoofNPSVariables.lvlib\\ST-11_S"(w354) -> ()  [unwired: 1 in, 1 out]
        n197 = shared-variable "My Computer\\SpoofNPSVariables.lvlib\\ST-12-N_S"(w354) -> ()  [unwired: 1 in, 1 out]
        n198 = shared-variable "My Computer\\SpoofNPSVariables.lvlib\\ST-12-SE_S"(w354) -> ()  [unwired: 1 in, 1 out]
        n199 = shared-variable "My Computer\\SpoofNPSVariables.lvlib\\ST-12-SW_S"(w354) -> ()  [unwired: 1 in, 1 out]
        n200 = shared-variable "My Computer\\SpoofNPSVariables.lvlib\\ST-13_S"(w354) -> ()  [unwired: 1 in, 1 out]
        n201 = shared-variable "My Computer\\SpoofNPSVariables.lvlib\\ST-14-E_S"(w354) -> ()  [unwired: 1 in, 1 out]
        n202 = shared-variable "My Computer\\SpoofNPSVariables.lvlib\\ST-14-N_S"(w354) -> ()  [unwired: 1 in, 1 out]
        n203 = shared-variable "My Computer\\SpoofNPSVariables.lvlib\\ST-14-S_S"(w354) -> ()  [unwired: 1 in, 1 out]
        n204 = shared-variable "My Computer\\SpoofNPSVariables.lvlib\\ST-14-W_S"(w354) -> ()  [unwired: 1 in, 1 out]
        n205 = shared-variable "My Computer\\SpoofNPSVariables.lvlib\\AT-01_S"(w354) -> ()  [unwired: 1 in, 1 out]
        n206 = shared-variable "My Computer\\SpoofNPSVariables.lvlib\\AT-02_S"(w354) -> ()  [unwired: 1 in, 1 out]
        n207 = shared-variable "My Computer\\SpoofNPSVariables.lvlib\\FM-20_S"(w352) -> ()  [unwired: 1 in, 1 out]
        n208 = shared-variable "My Computer\\SpoofNPSVariables.lvlib\\FM-30_S"(w352) -> ()  [unwired: 1 in, 1 out]
        n209 = shared-variable "My Computer\\SpoofNPSVariables.lvlib\\FM-40_S"(w352) -> ()  [unwired: 1 in, 1 out]
        n210 = shared-variable "My Computer\\SpoofNPSVariables.lvlib\\FM-60_S"(w352) -> ()  [unwired: 1 in, 1 out]
        n211 = shared-variable "My Computer\\SpoofVFD_Variables.lvlib\\Pump Frequency_S"(w352) -> ()  [unwired: 1 in, 1 out]
        n212 = shared-variable "My Computer\\SpoofVFD_Variables.lvlib\\CTAH Frequency_S"(w352) -> ()  [unwired: 1 in, 1 out]
        n213 = shared-variable "My Computer\\SpoofVFD_Variables.lvlib\\TCHX Frequency_S"(w352) -> ()  [unwired: 1 in, 1 out]
        n214 = shared-variable "My Computer\\SpoofCore_Variables.lvlib\\Power Output_S"(w352) -> ()  [unwired: 1 in, 1 out]
        n215 = shared-variable "My Computer\\Core_Variables.lvlib\\Power Output On"() -> (w351:bool)  [unwired: 1 in, 1 out]
        n216 = shared-variable "My Computer\\VFD_Variables.lvlib\\Activate CTAH"() -> (w350:bool)  [unwired: 1 in, 1 out]
        n217 = shared-variable "My Computer\\VFD_Variables.lvlib\\Activate Pump"() -> (w348:bool)  [unwired: 1 in, 1 out]
        n218 = shared-variable "My Computer\\VFD_Variables.lvlib\\Activate TCHX"() -> (w349:bool)  [unwired: 1 in, 1 out]
        n219 = shared-variable "My Computer\\SpoofCore_Variables.lvlib\\Power Output On_S"(w351) -> ()  [unwired: 1 in, 1 out]
        n220 = shared-variable "My Computer\\SpoofVFD_Variables.lvlib\\Activate CTAH_S"(w350) -> ()  [unwired: 1 in, 1 out]
        n221 = shared-variable "My Computer\\SpoofVFD_Variables.lvlib\\Activate TCHX_S"(w349) -> ()  [unwired: 1 in, 1 out]
        n222 = shared-variable "My Computer\\SpoofVFD_Variables.lvlib\\Activate Pump_S"(w348) -> ()  [unwired: 1 in, 1 out]
      }
    }
    n223 = shared-variable "My Computer\\RemoteVIVariables.lvlib\\Spoof Enabled"("Spoof Enabled") -> ()  [unwired: 1 in, 1 out]
    n224 = Build Array(w131, w130, w129, w128) -> (w127:sgl[])
    n225 = Build Array(w124, w123, w122, w121) -> (w120:sgl[])
    n226 = Build Array(w45, w41) -> (w86:sgl[])
    n227 = Build Array(w88, w44) -> (w89:sgl[])
    n228 = case shown="False" "Load Power Profile" {
      tunnel: [w371 w372] -> w65
      tunnel: w66 -> [w371 _]
      frame False {
      }
      frame True {
        n229 = call-poly <vilib>:"Read Delimited Spreadsheet.vi"("file path (dialog if empty)"="Dyn. Power Profile File", "transpose? (F)"=TRUE, "delimiter (\\t)"="," ("delimiter (\\t)")) -> ("first row"=w372:dbl[])  [unwired: 7 in, 5 out]
      }
    }
    n230 = Subtract(x=w63, y=w64) -> (x-y=→"System Loop Time (ms)":u32)
    n231 = To Double Precision Float(number=w86) -> (double precision float=w87:dbl[])
    n232 = To Double Precision Float(number=w127) -> (double precision float=w126:dbl[])
    n233 = To Double Precision Float(number=w120) -> (double precision float=w125:dbl[])
    n234 = To Double Precision Float(number=w89) -> (double precision float=w90:dbl[])
    n235 = call-poly <vilib>:"Mean.vi"("X"=w87) -> ("mean"=→"Heater Inlet":dbl)  [unwired: 1 out]
    n236 = call-poly <vilib>:"Mean.vi"("X"=w126) -> ("mean"=w47:dbl)  [unwired: 1 out]
    n237 = call-poly <vilib>:"Mean.vi"("X"=w125) -> ("mean"=w46:dbl)  [unwired: 1 out]
    n238 = call-poly <vilib>:"Mean.vi"("X"=w90) -> ("mean"=→"Heater Outlet":dbl)  [unwired: 1 out]
    n239 = To Single Precision Float(number=w47) -> (single precision float=→"CX-10":sgl)
    n240 = To Single Precision Float(number=w46) -> (single precision float=→"CX-11":sgl)
    n241 = shared-variable "My Computer\\NPSVariables.lvlib\\WT-20"() -> (→"WT-20":sgl)  [unwired: 1 in, 1 out]
    n242 = shared-variable "My Computer\\NPSVariables.lvlib\\BT-21"() -> (→"BT-21":sgl)  [unwired: 1 in, 1 out]
    n243 = shared-variable "My Computer\\NPSVariables.lvlib\\WT-22"() -> (→"WT-22":sgl)  [unwired: 1 in, 1 out]
    n244 = shared-variable "My Computer\\NPSVariables.lvlib\\BT-23"() -> (→"BT-23":sgl)  [unwired: 1 in, 1 out]
    n245 = shared-variable "My Computer\\NPSVariables.lvlib\\WT-24"() -> (→"WT-24":sgl)  [unwired: 1 in, 1 out]
    n246 = shared-variable "My Computer\\NPSVariables.lvlib\\BT-25"() -> (→"BT-25":sgl)  [unwired: 1 in, 1 out]
    n247 = shared-variable "My Computer\\NPSVariables.lvlib\\WT-26"() -> (→"WT-26":sgl)  [unwired: 1 in, 1 out]
    n248 = shared-variable "My Computer\\NPSVariables.lvlib\\BT-27"() -> (→"BT-27":sgl)  [unwired: 1 in, 1 out]
    n249 = shared-variable "My Computer\\NPSVariables.lvlib\\WT-28"() -> (→"WT-28":sgl)  [unwired: 1 in, 1 out]
    n250 = shared-variable "My Computer\\NPSVariables.lvlib\\BT-29"() -> (→"BT-29":sgl)  [unwired: 1 in, 1 out]
    n251 = shared-variable "My Computer\\Core_Variables.lvlib\\Shutdown"("Shutdown") -> ()  [unwired: 1 in, 1 out]
    n252 = shared-variable "My Computer\\RemoteVIVariables.lvlib\\Write Connection"() -> (w28:bool)  [unwired: 1 in, 1 out]
    n253 = shared-variable "My Computer\\RemoteVIVariables.lvlib\\Read Connection"() -> (w27:bool)  [unwired: 1 in, 1 out]
    n254 = shared-variable "My Computer\\RemoteVIVariables.lvlib\\Chat Connection"() -> (w29:bool)  [unwired: 1 in, 1 out]
    n255 = shared-variable "My Computer\\Core_Variables.lvlib\\Input Power Profile Array"(w65) -> ()  [unwired: 1 in, 1 out]
    n256 = shared-variable "My Computer\\DAQ_Variables.lvlib\\Flow Data?"("Flow Data?") -> ()  [unwired: 1 in, 1 out]
    n257 = shared-variable "My Computer\\Core_Variables.lvlib\\Loop Period"() -> (→"Loop Period [ms]":i64)  [unwired: 1 in, 1 out]
    n258 = shared-variable "My Computer\\Core_Variables.lvlib\\Output Voltage 1"() -> (→"Output Voltage 1 [V]":dbl)  [unwired: 1 in, 1 out]
    n259 = shared-variable "My Computer\\Core_Variables.lvlib\\Output Current 1"() -> (→"Output Current 1 [A]":dbl)  [unwired: 1 in, 1 out]
    n260 = shared-variable "My Computer\\Core_Variables.lvlib\\Output Voltage 2"() -> (→"Output Voltage 2 [V]":dbl)  [unwired: 1 in, 1 out]
    n261 = shared-variable "My Computer\\Core_Variables.lvlib\\Output Current 2"() -> (→"Output Current 2 [A]":dbl)  [unwired: 1 in, 1 out]
    n262 = shared-variable "My Computer\\Core_Variables.lvlib\\Power Input Signal"() -> (→"Power Input Signal [W]":sgl)  [unwired: 1 in, 1 out]
    n263 = shared-variable "My Computer\\Core_Variables.lvlib\\Power Output"() -> (→"Power [W]":sgl)  [unwired: 1 in, 1 out]
    n264 = shared-variable "My Computer\\Core_Variables.lvlib\\Profile Step"() -> (→"Profile Step":i32)  [unwired: 1 in, 1 out]
    n265 = Build Array(w29, w28, w27) -> (w26:bool[])
    n266 = And Array Elements(Boolean array=w26) -> (logical AND=→"Server Connection":bool)
    n267 = shared-variable "My Computer\\NPSVariables.lvlib\\BT-30"() -> (→"BT-30":sgl)  [unwired: 1 in, 1 out]
    n268 = shared-variable "My Computer\\NPSVariables.lvlib\\WT-31"() -> (→"WT-31":sgl)  [unwired: 1 in, 1 out]
    n269 = shared-variable "My Computer\\NPSVariables.lvlib\\BT-32"() -> (→"BT-32":sgl)  [unwired: 1 in, 1 out]
    n270 = shared-variable "My Computer\\NPSVariables.lvlib\\WT-33"() -> (→"WT-33":sgl)  [unwired: 1 in, 1 out]
    n271 = shared-variable "My Computer\\NPSVariables.lvlib\\BT-34"() -> (→"BT-34":sgl)  [unwired: 1 in, 1 out]
    n272 = shared-variable "My Computer\\NPSVariables.lvlib\\WT-35"() -> (→"WT-35":sgl)  [unwired: 1 in, 1 out]
    n273 = shared-variable "My Computer\\NPSVariables.lvlib\\WT-40"() -> (w72:sgl)  [unwired: 1 in, 1 out]
    "WT-40" <- w72
    n274 = shared-variable "My Computer\\NPSVariables.lvlib\\BT-41"() -> (w71:sgl)  [unwired: 1 in, 1 out]
    "BT-41" <- w71
    n275 = shared-variable "My Computer\\NPSVariables.lvlib\\WT-42"() -> (w74:sgl)  [unwired: 1 in, 1 out]
    "WT-42" <- w74
    n276 = shared-variable "My Computer\\NPSVariables.lvlib\\BT-43"() -> (w73:sgl)  [unwired: 1 in, 1 out]
    "BT-43" <- w73
    n277 = Build Array(w73, w74) -> (w79:sgl[])
    n278 = Build Array(w71, w72) -> (w76:sgl[])
    n279 = shared-variable "My Computer\\NPSVariables.lvlib\\BT-60"() -> (→"BT-60":sgl)  [unwired: 1 in, 1 out]
    n280 = shared-variable "My Computer\\NPSVariables.lvlib\\WT-61"() -> (→"WT-61":sgl)  [unwired: 1 in, 1 out]
    n281 = shared-variable "My Computer\\NPSVariables.lvlib\\WT-62"() -> (→"WT-62":sgl)  [unwired: 1 in, 1 out]
    n282 = shared-variable "My Computer\\NPSVariables.lvlib\\BT-63"() -> (→"BT-63":sgl)  [unwired: 1 in, 1 out]
    n283 = shared-variable "My Computer\\NPSVariables.lvlib\\WT-64"() -> (→"WT-64":sgl)  [unwired: 1 in, 1 out]
    n284 = shared-variable "My Computer\\NPSVariables.lvlib\\BT-65"() -> (→"BT-65":sgl)  [unwired: 1 in, 1 out]
    n285 = shared-variable "My Computer\\NPSVariables.lvlib\\BT-66"() -> (→"BT-66":sgl)  [unwired: 1 in, 1 out]
    n286 = shared-variable "My Computer\\NPSVariables.lvlib\\WT-67"() -> (→"WT-67":sgl)  [unwired: 1 in, 1 out]
    n287 = To Double Precision Float(number=w79) -> (double precision float=w80:dbl[])
    n288 = To Double Precision Float(number=w76) -> (double precision float=w77:dbl[])
    n289 = call-poly <vilib>:"Mean.vi"("X"=w80) -> ("mean"=→"CTAH Inlet":dbl)  [unwired: 1 out]
    n290 = call-poly <vilib>:"Mean.vi"("X"=w77) -> ("mean"=→"CTAH Outlet":dbl)  [unwired: 1 out]
    n291 = shared-variable "My Computer\\NPSVariables.lvlib\\ST-10"() -> (→"ST-10":sgl)  [unwired: 1 in, 1 out]
    n292 = shared-variable "My Computer\\NPSVariables.lvlib\\ST-11"() -> (→"ST-11":sgl)  [unwired: 1 in, 1 out]
    n293 = shared-variable "My Computer\\NPSVariables.lvlib\\ST-12-N"() -> (→"N":sgl)  [unwired: 1 in, 1 out]
    n294 = shared-variable "My Computer\\NPSVariables.lvlib\\ST-12-SE"() -> (→"SE":sgl)  [unwired: 1 in, 1 out]
    n295 = shared-variable "My Computer\\NPSVariables.lvlib\\ST-12-SW"() -> (→"SW":sgl)  [unwired: 1 in, 1 out]
    n296 = shared-variable "My Computer\\NPSVariables.lvlib\\ST-13"() -> (→"ST-13":sgl)  [unwired: 1 in, 1 out]
    n297 = shared-variable "My Computer\\NPSVariables.lvlib\\ST-14-N"() -> (→"N":sgl)  [unwired: 1 in, 1 out]
    n298 = shared-variable "My Computer\\NPSVariables.lvlib\\ST-14-E"() -> (→"E":sgl)  [unwired: 1 in, 1 out]
    n299 = shared-variable "My Computer\\NPSVariables.lvlib\\ST-14-S"() -> (→"S":sgl)  [unwired: 1 in, 1 out]
    n300 = shared-variable "My Computer\\NPSVariables.lvlib\\ST-14-W"() -> (→"W":sgl)  [unwired: 1 in, 1 out]
    n301 = shared-variable "My Computer\\NPSVariables.lvlib\\AT-01"() -> (→"AT-01":sgl)  [unwired: 1 in, 1 out]
    n302 = shared-variable "My Computer\\NPSVariables.lvlib\\AT-02"() -> (→"AT-02":sgl)  [unwired: 1 in, 1 out]
    n303 = shared-variable "My Computer\\NPSVariables.lvlib\\FM-20"() -> (→"DHX Primary Flow\n\n\nFM-20 [kg/s]":sgl)  [unwired: 1 in, 1 out]
    n304 = shared-variable "My Computer\\NPSVariables.lvlib\\FM-30"() -> (→"Bypass Flow\n\n\nFM-30 [kg/s]":sgl)  [unwired: 1 in, 1 out]
    n305 = shared-variable "My Computer\\NPSVariables.lvlib\\FM-40"() -> (→"Primary Flow\n\n\nFM-40 [kg/s]":sgl)  [unwired: 1 in, 1 out]
    n306 = shared-variable "My Computer\\NPSVariables.lvlib\\FM-60"() -> (→"DRACS Flow\n\n\nFM-60 [kg/s]":sgl)  [unwired: 1 in, 1 out]
    n307 = shared-variable "My Computer\\VFD_Variables.lvlib\\Pump Frequency"() -> (→"Frequency [Hz]":sgl)  [unwired: 1 in, 1 out]
    n308 = shared-variable "My Computer\\VFD_Variables.lvlib\\CTAH Frequency"() -> (→"Frequency [Hz] 3":sgl)  [unwired: 1 in, 1 out]
    n309 = shared-variable "My Computer\\VFD_Variables.lvlib\\TCHX Frequency"() -> (→"Frequency [Hz]":sgl)  [unwired: 1 in, 1 out]
    n310 = local read "Heater Outlet"() -> (w81:dbl)
    n311 = local read "CTAH Outlet"() -> (w69:dbl)
    n312 = local read "Power [W]"() -> (→"Power Output":sgl)
    n313 = local read "Heater Inlet"() -> (w82:dbl)
    n314 = local read "CTAH Inlet"() -> (w68:dbl)
    n315 = Bundle("Heater Inlet"=w82, "Heater Outlet"=w81) -> (→"Core Temperatures":cluster{"Heater Inlet":dbl, "Heater Outlet":dbl})  [unwired: 1 in]
    n316 = Bundle("CTAH Outlet"=w69, "CTAH Inlet"=w68) -> (→"CTAH Temperatures":cluster{"CTAH Outlet":dbl, "CTAH Inlet":dbl})  [unwired: 1 in]
    n317 = shared-variable "My Computer\\DAQ_Variables.lvlib\\SysFluidTemps"() -> (w56:sgl[])  [unwired: 1 in, 1 out]
    n318 = shared-variable "My Computer\\DAQ_Variables.lvlib\\SysSurfTemps"() -> (w58:sgl[])  [unwired: 1 in, 1 out]
    n319 = shared-variable "My Computer\\DAQ_Variables.lvlib\\SysFlowRates"() -> (w40:sgl[])  [unwired: 1 in, 1 out]
    n320 = shared-variable "My Computer\\SpoofDAQ_Variables.lvlib\\SysFlowRates_S"(w40) -> ()  [unwired: 1 in, 1 out]
    n321 = Less?(x=w58, y=sgl 250.0) -> (x < y?=w60:bool[])
    n322 = Less?(x=w56, y=sgl 130.0) -> (x < y?=w54:bool[])
    n323 = Less?(x=w40, y=sgl 0.2) -> (x < y?=w53:bool[])
    n324 = shared-variable "My Computer\\VFD_Variables.lvlib\\CTAH Operating Case"("CTAH Operation Mode") -> ()  [unwired: 1 in, 1 out]
    n325 = shared-variable "My Computer\\VFD_Variables.lvlib\\Pump Operating Case"("Pump Operation Mode") -> ()  [unwired: 1 in, 1 out]
    n326 = shared-variable "My Computer\\VFD_Variables.lvlib\\TCHX Operating Case"("TCHX Operation Mode") -> ()  [unwired: 1 in, 1 out]
    n327 = Build Array (concatenate)(w60, w54, w53) -> (w61:bool[])
    n328 = shared-variable "My Computer\\VFD_Variables.lvlib\\Activate CTAH"("ACTIVATE - CTAH") -> ()  [unwired: 1 in, 1 out]
    n329 = shared-variable "My Computer\\VFD_Variables.lvlib\\Activate Pump"("ACTIVATE - PUMP") -> ()  [unwired: 1 in, 1 out]
    n330 = shared-variable "My Computer\\VFD_Variables.lvlib\\Activate TCHX"("ACTIVATE - TCHX") -> ()  [unwired: 1 in, 1 out]
    n331 = And Array Elements(Boolean array=w61) -> (logical AND=→"System Safe":bool)
    n332 = shared-variable "My Computer\\VFD_Variables.lvlib\\GS1 Stop"("VFD Stop") -> ()  [unwired: 1 in, 1 out]
    "Numeric" <- w30
  }
  n333 = call "Remote VI Close.vi"("reference"=w6) -> ()  [unwired: 10 in, 1 out]
  n334 = call "Remote VI Close.vi"("reference"=w5) -> ()  [unwired: 10 in, 1 out]
  n335 = shared-variable "My Computer\\RemoteVIVariables.lvlib\\Stop Broadcasting"(w1) -> ()  [unwired: 1 in, 1 out]
  n336 = shared-variable "My Computer\\RemoteVIVariables.lvlib\\Spoof Enabled"(w1) -> ()  [unwired: 1 in, 1 out]
  n337 = shared-variable "My Computer\\RemoteVIVariables.lvlib\\Stop Chat"(w1) -> ()  [unwired: 1 in, 1 out]
  n338 = call "Remote VI Close.vi"("reference"=w2) -> ()  [unwired: 10 in, 1 out]
  n339 = shared-variable "My Computer\\RemoteVIVariables.lvlib\\Stop Reading"(w1) -> ()  [unwired: 1 in, 1 out]
